vi "Get Msg Attributes.vi"(11 "Actor Create in":refnum<class "Actor Create.lvclass">) -> (1 "Nest Alias":string, 2 "Nest Actor":refnum<class "Actor.lvclass">)   [LabVIEW 2021, in "Actor Create.lvlib" / "Actor Create.lvclass"]
uses:
  Actor Create.lvclass
  LVCAM/Actor/Actor.lvclass
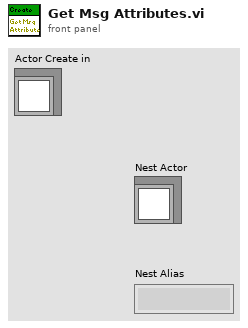
[diagram p1: front panel]
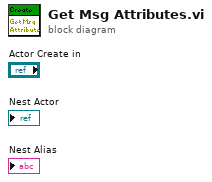
[diagram p0: block diagram]
diagram:
